vi "set_parameters.vi"(8 "error in (no error)":errorcluster) -> (0 "error out (no error)":errorcluster)   [LabVIEW 2019, in "Glaz.lvclass"]
uses:
  Glaz.lvclass
  <userlib>/GlazLabView/GlazLib.lvlib
panel:
  in  "script file":path
  in  "continue":bool
  in  "Integration\nTime [us]":i32=2
  in  "HW Averaging":T1(ring)
  in  "Trigger Mode":enum16{"External", "Internal", "Burst"}(ring)=enum."Internal"
  in  "Integration Mode":enum16{"PulseSync", "TimeFill"}(ring)
  in  "scanCount":i32=500
  in  "trig delay":i32
  in  "internal freq":dbl=3000.0
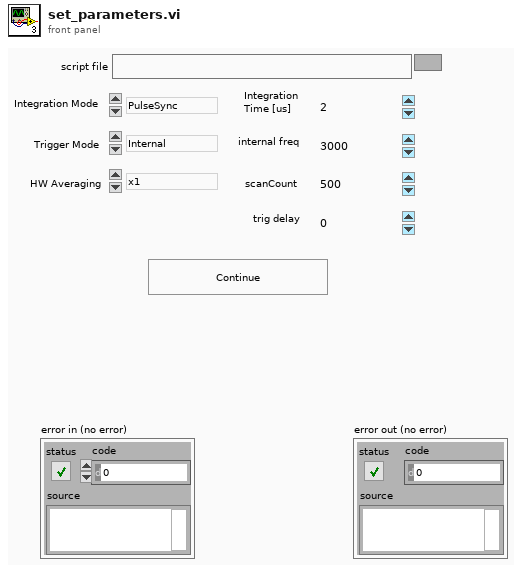
[diagram p1: front panel]
types:
  T1 = enum16{"x1", "x2", "x4", "x8", "x16", "x32", "x64", "x128", "x256"}
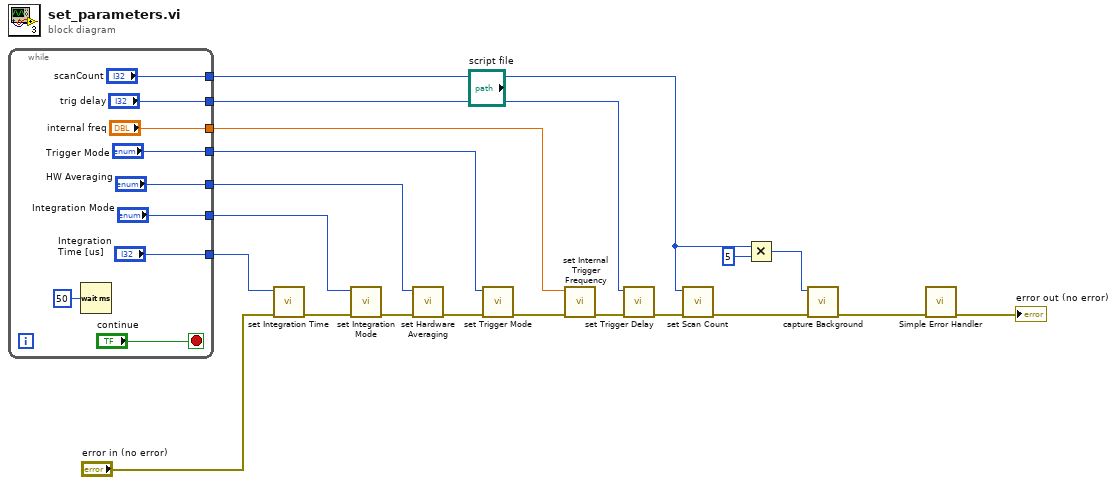
[diagram p0: block diagram]
diagram:
  n1 = while {
    tunnel: ["internal freq"] -> w12
    tunnel: ["trig delay"] -> w11
    tunnel: ["Integration Mode"] -> w10
    tunnel: ["Trigger Mode"] -> w9
    tunnel: ["HW Averaging"] -> w8
    tunnel: ["Integration\nTime [us]"] -> w7
    tunnel: ["scanCount"] -> w5
    stop <- "continue" stop-if-true
    n2 = Wait (ms)(milliseconds to wait=u32 50) -> ()  [unwired: 1 out]
  }
  n3 = call <userlib>:"set Integration Time.vi"("error in (no error)"="error in (no error)", "us"=w7) -> ("error out"=w14:errorcluster)  [unwired: 8 in, 1 out]
  n4 = call <userlib>:"set Integration Mode.vi"("error in (no error)"=w14, "mode"=w10) -> ("error out"=w15:errorcluster)  [unwired: 8 in, 1 out]
  n5 = call <userlib>:"set Hardware Averaging.vi"("error in (no error)"=w15, "averaging"=w8) -> ("error out"=w16:errorcluster)  [unwired: 8 in, 1 out]
  n6 = call <userlib>:"set Trigger Mode.vi"("error in (no error)"=w16, "mode"=w9) -> ("error out"=w17:errorcluster)  [unwired: 8 in, 1 out]
  n7 = call <userlib>:"set Internal Trigger Frequency.vi"("error in (no error)"=w17, "Hz"=w12) -> ("error out"=w18:errorcluster)  [unwired: 8 in, 1 out]
  n8 = call <userlib>:"set Trigger Delay.vi"("error in (no error)"=w18, "us"=w11) -> ("error out"=w19:errorcluster)  [unwired: 8 in, 1 out]
  n9 = call <userlib>:"set Scan Count.vi"("error in (no error)"=w19, "scanCount"=w5) -> ("error out"=w6:errorcluster)  [unwired: 8 in, 1 out]
  n10 = Multiply(x=w5, y=5) -> (x*y=w3:i32)
  n11 = call <userlib>:"capture Background.vi"("error in (no error)"=w6, "scanCount"=w3) -> ("error out"=w2:errorcluster)  [unwired: 8 in, 1 out]
  n12 = call <vilib>:"Simple Error Handler.vi"("error in (no error)"=w2) -> ("error out"=→"error out (no error)":errorcluster)  [unwired: 4 in, 4 out]
